vi "Arcade Drive.vi"(10 "Y Axis":dbl, 11 "X Axis":dbl) -> (2 "Left Motor Value":dbl, 3 "Right Motor Value":dbl)   [LabVIEW 2012]
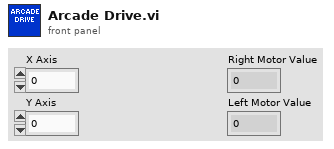
[diagram p1: front panel]
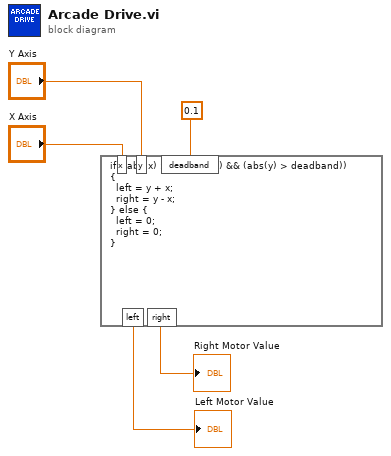
[diagram p0: block diagram]
diagram:
  n1 = formula code="if ((abs(x) > deadband) && (abs(y) > deadband))\n{\n  left = y + x;\n  right = y - x;\n} else {\n  left = 0;\n  right = 0;\n}"("x"="X Axis", "y"="Y Axis", "deadband"=0.1 ("input variable")) -> ("left"=→"Left Motor Value":dbl, "right"=→"Right Motor Value":dbl)
